vi "Unreserve.vi"(8 "error in (no error)":errorcluster, 9 "Sequence Parameters in":variant, 11 "Example Step One in":refnum<class "Example Step One.lvclass">) -> (0 "error out":errorcluster, 1 "Sequence Parameters out":variant, 3 "Example Step One out":refnum<class "Example Step One.lvclass">)   [LabVIEW 2015, in "Mediator.lvlib" / "Example Step One.lvclass"]
doc: "This unreserves any resources used by this step."
uses:
  Example Step One.lvclass
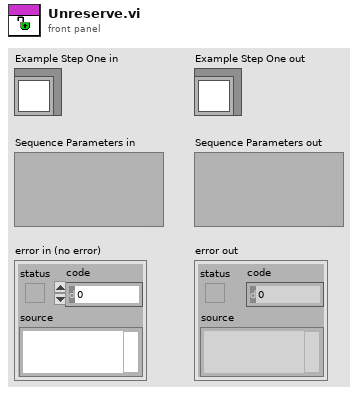
[diagram p1: front panel]
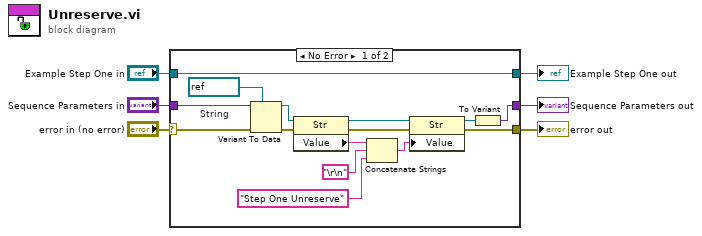
[diagram p0: block diagram]
diagram:
  n1 = case shown="No Error" "error in (no error)" {
    selector: "error in (no error)" -> [w20 w23]
    tunnel: [w7 w23] -> w1
    tunnel: "Sequence Parameters in" -> [w21 w22]
    tunnel: "Example Step One in" -> [w19 w24]
    tunnel: [w19 w24] -> w3
    tunnel: [w11 w22] -> w2
    frame No Error {
      w18 = refnum<vi> refnum  # String
      n2 = Variant To Data(error in=w20, type=w18, Variant=w21) -> (data=w17:refnum<vi>, error out=w9:errorcluster)
      n3 = property class="Str"(reference=w17, error in=w9) -> (reference out=w13:refnum<vi>, error out=w8:errorcluster, "Value"=w16:string)
      n4 = Concatenate Strings(w16, "\r\n", "Step One Unreserve" ("string")) -> (w12:string)
      n5 = property class="Str"(reference=w13, error in=w8, "Value"=w12) -> (reference out=w10:refnum<vi>, error out=w7:errorcluster)
      n6 = To Variant(anything=w10) -> (Variant=w11:variant)
    }
    frame Error {
    }
  }
  "error out" <- w1
  "Example Step One out" <- w3
  "Sequence Parameters out" <- w2
